vi "sendRunSingleScript.vi"(8 "error in (no error)":errorcluster, 9 "HWLoop":bool, 10 "Path":path, 11 "ExperimentControlEvents in":refnum<class "ExperimentControlEvents.lvclass">) -> (0 "error out":errorcluster, 3 "ExperimentControlEvents out":refnum<class "ExperimentControlEvents.lvclass">)   [LabVIEW 2011, in "Views.lvlib" / "ExperimentControl.lvlib" / "ExperimentControlEvents.lvclass"]
uses:
  ExperimentControlEvents.lvclass
  ExperimentControlEvents.lvclass/ExperimentControlEvents.ctl
  Events/Event.lvclass
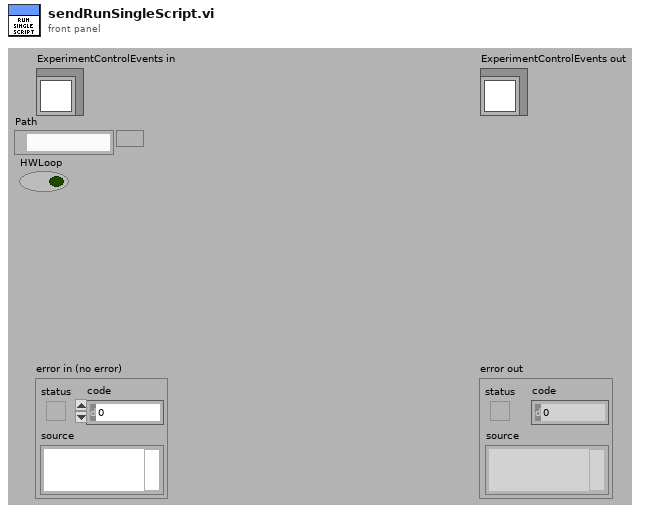
[diagram p1: front panel]
types:
  T1 = enum16{"close", "stopRunning", "runSingleScript", "runExperiment", "runExperimentScript"}
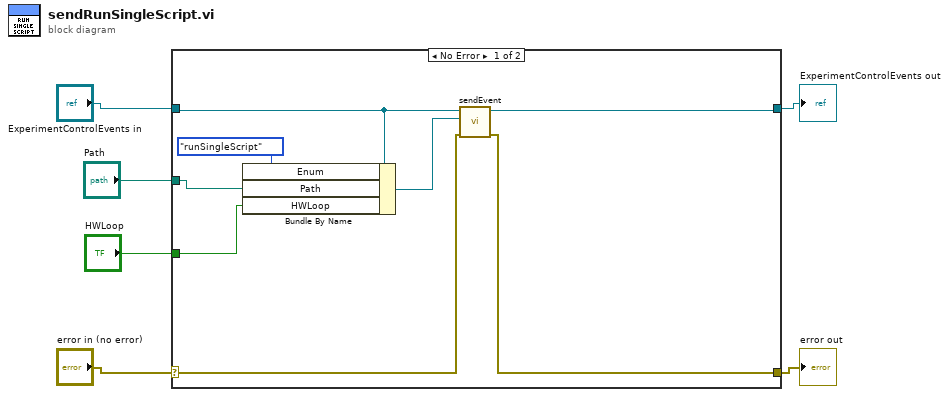
[diagram p0: block diagram]
diagram:
  n1 = case shown="No Error" "error in (no error)" {
    selector: "error in (no error)" -> [w10 w16]
    tunnel: [w9 w16] -> w3
    tunnel: [w14 w15] -> w6
    tunnel: "ExperimentControlEvents in" -> [w13 w15]
    tunnel: "Path" -> [w8 _]
    tunnel: "HWLoop" -> [w7 _]
    frame No Error {
      n2 = Bundle By Name(cluster=w13, "Enum"=T1."runSingleScript", "Path"=w8, "HWLoop"=w7) -> (w12:refnum<class "ExperimentControlEvents.lvclass">)
      n3 = call "sendEvent.vi"("error in (no error)"=w10, "data"=w12, "Event in"=w13) -> ("error out"=w9:errorcluster, "Event out"=w14:refnum<class "ExperimentControlEvents.lvclass">)  [unwired: 7 in]
    }
    frame Error {
    }
  }
  "error out" <- w3
  "ExperimentControlEvents out" <- w6
